vi "Frontend FPP.vi"() -> ()   [LabVIEW 2016]
panel:
  in  "Gate 2":T1={"Gate Start"=0.0, "Gate Stop"=2.0, "Gate Step (linear only)"=1.0, "Gate Compliance"=0.0001, "Gate PComp"=0.0, "Range mode"=0, "Range"=6} {"Range" max=11 scale=0.0..11.0; "Range mode" items=["Auto", "Limited", "Fixed"]; "Gate PComp" format="%^.2e"; "Gate Compliance" format="%^.2e"; "Gate Step (linear only)" format="%^.4e"; "Gate Stop" format="%^.4e"; "Gate Start" format="%^.4e"}
  in  "Drain":T2={"Drain Start"=0.0, "Drain Stop"=2.0, "Drain Compliance"=0.0001, "Drain Step"=1.0, "Drain PComp"=0.0, "Range mode"=0, "Range"=6} {"Range" max=11 scale=0.0..11.0; "Range mode" items=["Auto", "Limited", "Fixed"]; "Drain PComp" format="%^.2e"; "Drain Step" format="%^.4e"; "Drain Compliance" format="%^.2e"; "Drain Stop" format="%^.4e"; "Drain Start" format="%^.4e"}
  in  "Gate":T3={"Gate Start"=0.0, "Gate Stop"=2.0, "Gate Step"=1.0, "Gate Compliance"=0.0001, "Gate PComp"=0.0, "Range mode"=0, "Range"=6} {"Range" max=11 scale=0.0..11.0; "Range mode" items=["Auto", "Limited", "Fixed"]; "Gate PComp" format="%^.2e"; "Gate Compliance" format="%^.2e"; "Gate Step" format="%^.4e"; "Gate Stop" format="%^.4e"; "Gate Start" format="%^.4e"}
  in  "Drain 2":T4={"Drain Start"=0.0, "Drain Stop"=2.0, "Drain Compliance"=0.0001, "Drain Step (linear only)"=1.0, "Drain PComp"=0.0, "Range mode"=0, "Range"=6} {"Range" max=11 scale=0.0..11.0; "Range mode" items=["Auto", "Limited", "Fixed"]; "Drain PComp" format="%^.2e"; "Drain Step (linear only)" format="%^.4e"; "Drain Compliance" format="%^.2e"; "Drain Stop" format="%^.4e"; "Drain Start" format="%^.4e"}
  in  "Timings":T5={"integration time"=0, "Short/Long integration time"=0.00064, "hold time (sec)"=0.0, "delay time (sec)"=0.0, "Step Time (0 disables)"=0.0, "sweep method"=0, "Pulse period"=0.005, "Base voltage"=0.0, "Pulse width"=0.0005} {"Pulse width" min=0.0005 max=0.1 step=0.0001 format="%.4f"; "Base voltage" format="%^.4e"; "Pulse period" min=0.005 max=1.0 step=0.0001 format="%.4f"; "sweep method" items=["Continuous", "Pulsed"]; "Step Time (0 disables)" format="%.2f"; "delay time (sec)" format="%.4f"; "hold time (sec)" format="%.4f"; "Short/Long integration time" format="%^.0e"; "integration time" scale=0.0..2.0}
  in  "Panel controls":T6={"Emergency Stop"=refnum, "OutputGraph Max"=1e-05, "Text/Graph (text=false)"=FALSE} {"OutputGraph Max" format="%.2e"}
  in  "Panel Controls":T7={"Emergency Stop"=refnum, "TransGraph Max"=1e-05, "Text/Graph (text=false)"=FALSE} {"TransGraph Max" format="%.2e"}
  in  "Tab Control":enum32{"Characteristics", "Other parameters"}(tab)
  out "XY Graph 2":cluster{"Y data in":dbl[], "X data in":dbl[]}[](graph)
  in  "Integration time (long)":dbl=0.32 min=0.04 max=2.0 step=0.02 format="%.2f"
  in  "Integration time (short)":dbl=0.00064 min=8e-05 max=0.00192 step=8e-05 format="%^.0e"
  in  "Drain Range":u8(slide)=6 max=11 scale=0.0..11.0
  in  "Drain Range mode":u16(ring) items=["Auto", "Limited", "Fixed"]
  in  "Gate Range":u8(slide)=6 max=11 scale=0.0..11.0
  in  "Gate Range mode":u16(ring) items=["Auto", "Limited", "Fixed"]
  in  "Sampling mode":u32(slide) scale=0.0..4.0
  in  "Number of Samples":i32=500 min=0 step=1
  in  "Time":dbl=240.0 min=0.0 format="%.2f"
  in  "Drain":dbl=-10.0 min=-100.0 max=100.0 format="%.2f"
  in  "Gate":dbl=-60.0 min=-100.0 max=100.0 format="%.2f"
  in  "sweep method":u16(ring) items=["Continuous", "Pulsed"]
  out "Id":dbl format="%.2e"
  out "Ig":dbl format="%.2e"
  in  "Sweep Start":bool caption="Sweep start"
  in  "Interrupt run":bool
  in  "Running":bool
  out "Path":path
  in  "integration time":u32(slide)=1 max=2 step=1 scale=0.0..2.0
  in  "sweep mode":u16(ring)=1 items=["Single", "Double"]
  in  "Transfer Start":bool
  in  "Output Start":bool
  in  "Drain: Step":dbl=-1.0 min=-100.0 max=100.0 format="%.2f"
  in  "Drain: Stop":dbl=-60.0 min=-100.0 max=100.0 format="%.2f"
  in  "Drain:Start":dbl min=-100.0 max=100.0 format="%.2f"
  in  "Gate: Step":dbl=-20.0 min=-100.0 max=100.0 format="%.2f"
  in  "Gate: Stop":dbl=-60.0 min=-100.0 max=100.0 format="%.2f"
  in  "Gate: Start":dbl min=-100.0 max=100.0 format="%.2f"
  out "XY Graph":cluster{"Y data in":dbl[], "X data in":dbl[]}[](graph)
  in  "Drain: Compliance":dbl=0.001 min=1e-12 max=0.02 format="%.8f"
  in  "Gate: Compliance":dbl=0.001 min=1e-12 max=0.02 format="%.8f"
  in  "Drain: Step":dbl=-5.0 min=-100.0 max=100.0 format="%.2f"
  in  "Drain: Stop":dbl=-10.0 min=-100.0 max=100.0 format="%.2f"
  in  "Drain:Start":dbl=-5.0 min=-100.0 max=100.0 format="%.2f"
  in  "Gate: Step":dbl=-1.0 min=-100.0 max=100.0 format="%.2f"
  in  "Gate: Stop":dbl=-60.0 min=-100.0 max=100.0 format="%.2f"
  in  "Gate: Start":dbl=10.0 min=-100.0 max=100.0 format="%.2f"
  in  "Pulse width":dbl=0.0005 min=0.0005 max=0.1 step=0.0001 format="%.4f"
  in  "Base voltage":dbl min=-100.0 max=100.0 format="%.2f"
  in  "Pulse period":dbl=0.005 min=0.005 max=1.0 step=0.0001 format="%.4f"
  in  "Drain Power Compliance":dbl min=0.0 max=1.0 format="%.2f"
  in  "Gate Power\nCompliance":dbl min=0.0 max=1.0 format="%.2f"
  in  "OutputGraph Max":dbl=1e-05 format="%.2e"
  in  "TransGraph Max":dbl=1e-05 format="%.2e"
  in  "SPA Display":bool
  in  "Step delay /s":dbl min=0.0 max=1.0 format="%.2f"
  in  "hold time /s":dbl min=0.0 max=655.35 step=0.01 format="%.2f"
  in  "delay time /s":dbl min=0.0 max=65.535 step=0.0001 format="%.2f"
  in  "Decimal places in header":i8=1
  out "error out":errorcluster
  # "Transfer Characteristics"
  # "Stress Measurements"
  # "V"
  # "V"
  # "V"
  # "Gate"
  # "V"
  # "V"
  # "V"
  # "V"
  # "Drain"
  # "V"
  # "s"
  # "Output Characteristics"
  # "V"
  # "V"
  # "V"
  # "Gate"
  # "V"
  # "V"
  # "Drain"
  # "V"
  # "For Four Point Probe measurements ONLY!"
  # "SMU1 = Probe 1\nSMU2 = Drain\nSMU3 = Gate\nSMU4 = Probe 2\nVSU1 = Source"
  # "A"
  # "A"
  # "Vp1"
  # "Vp2"
  # "s"
  # "Pulsed mode settings"
  # "s"
  # "NOTE - THIS OVERRIDES THE COMPLIANCE VALUES!"
  # "A"
  # "A"
  # "Enter max power in Watts (max 1W)"
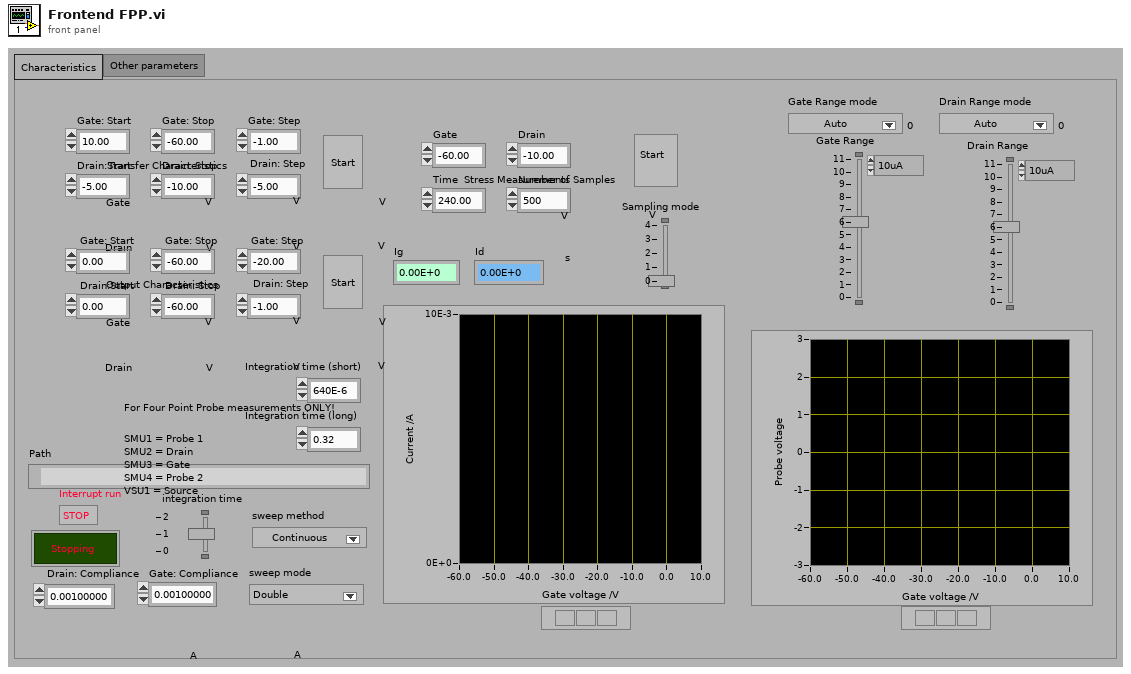
[diagram p1: front panel]
types:
  T1 = cluster{"Gate Start":dbl, "Gate Stop":dbl, "Gate Step (linear only)":dbl, "Gate Compliance":dbl, "Gate PComp":dbl, "Range mode":u16, "Range":u8}
  T2 = cluster{"Drain Start":dbl, "Drain Stop":dbl, "Drain Compliance":dbl, "Drain Step":dbl, "Drain PComp":dbl, "Range mode":u16, "Range":u8}
  T3 = cluster{"Gate Start":dbl, "Gate Stop":dbl, "Gate Step":dbl, "Gate Compliance":dbl, "Gate PComp":dbl, "Range mode":u16, "Range":u8}
  T4 = cluster{"Drain Start":dbl, "Drain Stop":dbl, "Drain Compliance":dbl, "Drain Step (linear only)":dbl, "Drain PComp":dbl, "Range mode":u16, "Range":u8}
  T5 = cluster{"integration time":u32, "Short/Long integration time":dbl, "hold time (sec)":dbl, "delay time (sec)":dbl, "Step Time (0 disables)":dbl, "sweep method":u16, "Pulse period":dbl, "Base voltage":dbl, "Pulse width":dbl}
  T6 = cluster{"Emergency Stop":refnum<vi>, "OutputGraph Max":dbl, "Text/Graph (text=false)":bool}
  T7 = cluster{"Emergency Stop":refnum<vi>, "TransGraph Max":dbl, "Text/Graph (text=false)":bool}
  T8 = cluster{"V2 Start":dbl, "V2 Step":dbl, "Number of points":i32}
  T9 = enum16{"open", "replace", "create", "open or create", "replace or create", "replace or create with confirmation"}
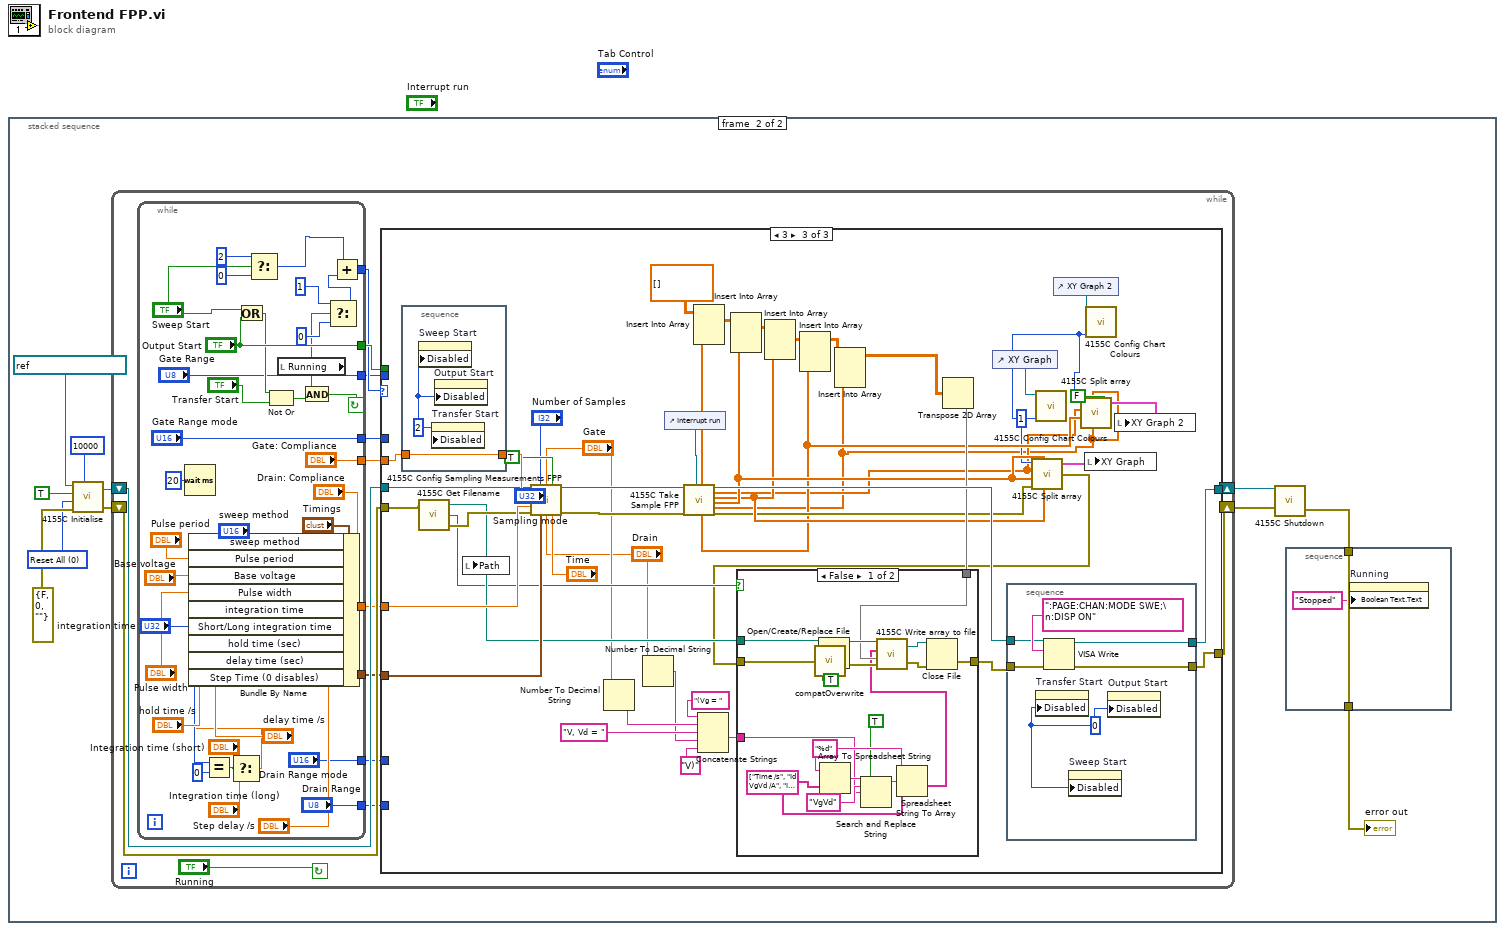
[diagram p0: block diagram]
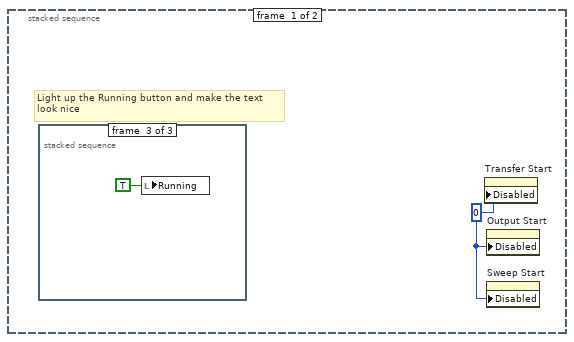
[diagram p2: hidden frame]
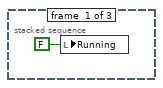
[diagram p3: hidden frame]
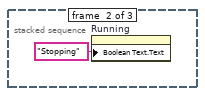
[diagram p4: hidden frame]
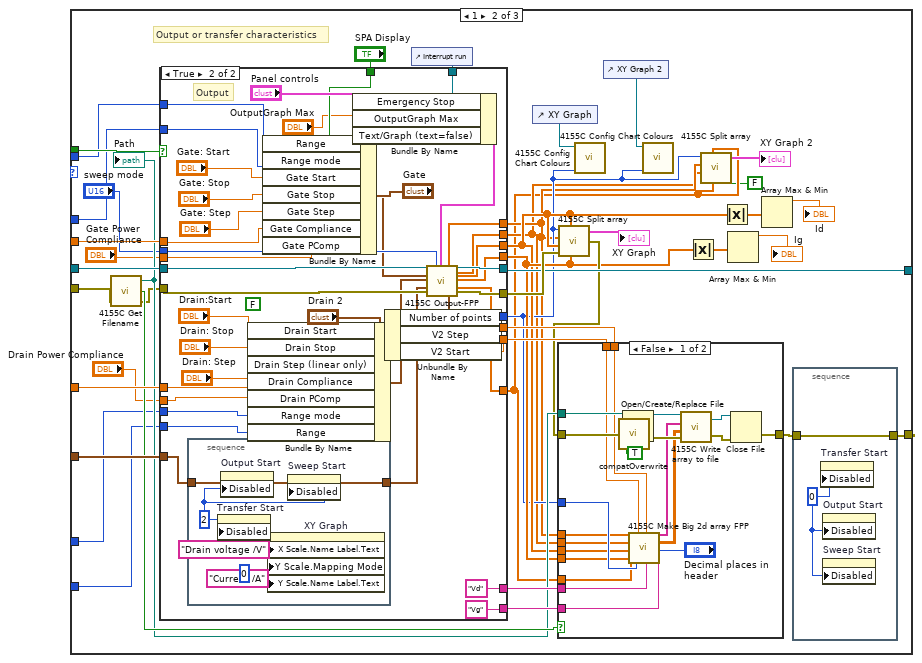
[diagram p6: hidden frame]
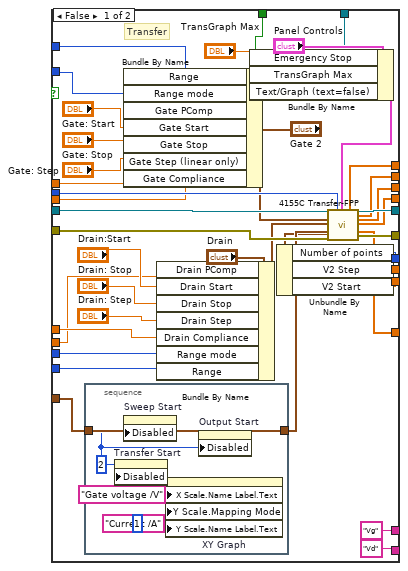
[diagram p8: hidden frame]
diagram:
  n1 = stacked-sequence {
    frame #0 {
      w1 = u8 0 ("Disabled")
      # "Light up the Running button and make the text\nlook nice"
      n2 = stacked-sequence {
        frame #0 {
          n3 = local write "Running"(FALSE ("Running")) -> ()
        }
        frame #1 {
          n4 = property on="Running" class="Bool (strict)"("Boolean Text.Text"="Stopping") -> ()  [unwired: 2 in, 2 out]
        }
        frame #2 {
          (unwired) FALSE ("Running")
          n5 = local write "Running"(TRUE ("Running")) -> ()
        }
      }
      n6 = property on="Transfer Start" class="Bool (strict)"("Disabled"=w1) -> ()  [unwired: 2 in, 2 out]
      n7 = property on="Output Start" class="Bool (strict)"("Disabled"=w1) -> ()  [unwired: 2 in, 2 out]
      n8 = property on="Sweep Start" class="Bool (strict)"("Disabled"=w1) -> ()  [unwired: 2 in, 2 out]
    }
    frame #1 {
      w11 = u16 0 items=["Reset All", "Partial reset"] ("Type of reset")
      n9 = call "4155C Initialise.vi"("VISA resource name in"=refnum<visa-resource-name> "GPIB0::14::INSTR", "Reset"=TRUE, "Type of reset"=w11, "error in (no error)"=errorcluster {"status"=FALSE, "code"=0, "source"=""}, "VISA Timeout Value"=u32 10000) -> ("VISA Resource Name out"=w10:refnum<visa-resource-name>, "error out"=w9:errorcluster)
      n10 = while {
        shift-left: w10 -> [w24]
        shift-right: [w26] -> w5
        shift-left: w9 -> [w25]
        shift-right: [w27] -> w6
        stop <- "Running" continue-if-true
        n11 = while {
          tunnel: ["Gate Range"] -> w16
          tunnel: ["Gate Range mode"] -> w17
          tunnel: ["Drain Range"] -> w18
          tunnel: ["Drain Range mode"] -> w19
          tunnel: ["Drain: Compliance"] -> w20
          tunnel: [w49] -> w21
          tunnel: ["Gate: Compliance"] -> w22
          tunnel: [w55] -> w23
          tunnel: ["Output Start"] -> w28
          stop <- w64 continue-if-true
          n12 = Wait (ms)(milliseconds to wait=u32 20) -> ()  [unwired: 1 out]
          n13 = Equal?(x="integration time", y=u32 0) -> (x = y?=w46:bool)
          n14 = Select(t="Integration time (short)", s=w46, f="Integration time (long)") -> (s? t:f=w43:dbl)
          n15 = Bundle By Name(cluster="Timings", "sweep method"="sweep method", "Pulse period"="Pulse period", "Base voltage"="Base voltage", "Pulse width"="Pulse width", "integration time"="integration time", "Short/Long integration time"=w43, "hold time (sec)"="hold time /s", "delay time (sec)"="delay time /s", "Step Time (0 disables)"="Step delay /s") -> (w49:T5)
          n16 = Or(x="Sweep Start", y="Output Start") -> (x .or. y?=w61:bool)
          n17 = Select(t=i8 2, s="Sweep Start", f=i8 0) -> (s? t:f=w31:i8)
          n18 = Not Or(1:"Transfer Start", 2:w61) -> (0:w63:bool)
          n19 = local read "Running"() -> (w58:bool)
          n20 = And(x=w58, y=w63) -> (x .and. y?=w64:bool)
          n21 = Select(t=i8 1, s=w58, f=i8 0) -> (s? t:f=w54:i8)
          n22 = Add(x=w31, y=w54) -> (x+y=w55:i8)
        }
        n23 = case shown="3" w23 {
          tunnel: w28 -> [_ w109 _]
          tunnel: w21 -> [_ w108 w266]
          tunnel: w22 -> [_ w107 w274]
          tunnel: w20 -> [_ w106 w270]
          tunnel: [w67 w97 w272] -> w27
          tunnel: [w66 w100 w273] -> w26
          tunnel: w25 -> [w67 w91 w261]
          tunnel: w24 -> [w66 w99 w260]
          tunnel: w19 -> [_ w81 _]
          tunnel: w18 -> [_ w80 _]
          tunnel: w17 -> [_ w79 _]
          tunnel: w16 -> [_ w78 _]
          frame 0, Default {
            # "Someone's deselected the running button so just shutdown..."
          }
          frame 1 {
            # "Output or transfer characteristics"
            n24 = call "4155C Get Filename.vi"("error in (no error)"=w91) -> ("error out"=w90:errorcluster, "cancelled"=w96:bool, "path"=w95:path)  [unwired: 2 in]
            "Path" <- w95
            n25 = control-ref of="Interrupt run"() -> (w92:refnum<vi>)
            n26 = case shown="True" w109 {
              tunnel: w99 -> [w161 w207]
              tunnel: w90 -> [w160 w206]
              tunnel: w108 -> [w164 w212]
              tunnel: w107 -> [w170 w219]
              tunnel: w106 -> [w175 w218]
              tunnel: "sweep mode" -> [w169 w217]
              tunnel: [w137 w185] -> w71
              tunnel: [w136 w184] -> w70
              tunnel: [w139 w183] -> w77
              tunnel: [w138 w182] -> w82
              tunnel: [w168 w216] -> w100
              tunnel: [w167 w215] -> w105
              tunnel: [w140 w188] -> w72
              tunnel: [w141 w187] -> w103
              tunnel: [w142 w186] -> w104
              tunnel: ["Vg" "Vd"] -> w102
              tunnel: ["Vd" "Vg"] -> w101
              tunnel: w92 -> [w158 w205]
              tunnel: "SPA Display" -> [w157 w203]
              tunnel: "Drain Power Compliance" -> [w153 w200]
              tunnel: "Gate Power\nCompliance" -> [w154 w199]
              tunnel: w81 -> [w145 w193]
              tunnel: w80 -> [w144 w192]
              tunnel: w79 -> [w146 w191]
              tunnel: w78 -> [w147 w190]
              tunnel: [w135 w181] -> w69
              frame False {
                # "Transfer"
                n27 = stacked-sequence {
                  tunnel: w164 -> [w179]
                  tunnel: [w179] -> w152
                  frame #0 {
                    w177 = u8 2 ("Disabled")
                    n28 = property on="Transfer Start" class="Bool (strict)"("Disabled"=w177) -> ()  [unwired: 2 in, 2 out]
                    n29 = property on="Sweep Start" class="Bool (strict)"("Disabled"=w177) -> ()  [unwired: 2 in, 2 out]
                    n30 = property on="XY Graph" class="XYGraph (strict)"("X Scale.Name Label.Text"="Gate voltage /V", "Y Scale.Mapping Mode"=u8 1, "Y Scale.Name Label.Text"="Current /A") -> ()  [unwired: 2 in, 2 out]
                    n31 = property on="Output Start" class="Bool (strict)"("Disabled"=w177) -> ()  [unwired: 2 in, 2 out]
                  }
                }
                n32 = Bundle By Name(cluster="Gate 2", "Range"=w147, "Range mode"=w146, "Gate PComp"=w154, "Gate Start"="Gate: Start", "Gate Stop"="Gate: Stop", "Gate Step (linear only)"="Gate: Step", "Gate Compliance"=w170) -> (w148:T1)
                n33 = Bundle By Name(cluster="Drain", "Drain PComp"=w153, "Drain Start"="Drain:Start", "Drain Stop"="Drain: Stop", "Drain Step"="Drain: Step", "Drain Compliance"=w175, "Range mode"=w145, "Range"=w144) -> (w150:T2)
                n34 = Bundle By Name(cluster="Panel Controls", "Emergency Stop"=w158, "TransGraph Max"="TransGraph Max", "Text/Graph (text=false)"=w157) -> (w155:T7)
                n35 = call "4155C Transfer-FPP.vi"("VISA resource name in"=w161, "Gate"=w148, "Drain"=w150, "Timings"=w152, "error in (no error)"=w160, "sweep mode"=w169, "Panel Controls"=w155) -> ("VG"=w137:dbl[], "Outparams"=w143:T8, "VISA Resource Name out"=w168:refnum<visa-resource-name>, "Vprobe2"=w136:dbl[], "ID"=w139:dbl[], "IG"=w138:dbl[], "Vprobe1"=w135:dbl[], "error out"=w167:errorcluster)  [unwired: 13 in]
                n36 = Unbundle By Name(w143) -> ("Number of points"=w140:i32, "V2 Step"=w141:dbl, "V2 Start"=w142:dbl)
              }
              frame True {
                (unwired) FALSE ("Logarithmic")
                # "Output"
                n37 = stacked-sequence {
                  tunnel: w212 -> [w225]
                  tunnel: [w225] -> w198
                  frame #0 {
                    w223 = u8 2 ("Disabled")
                    n38 = property on="Transfer Start" class="Bool (strict)"("Disabled"=w223) -> ()  [unwired: 2 in, 2 out]
                    n39 = property on="Output Start" class="Bool (strict)"("Disabled"=w223) -> ()  [unwired: 2 in, 2 out]
                    n40 = property on="XY Graph" class="XYGraph (strict)"("X Scale.Name Label.Text"="Drain voltage /V", "Y Scale.Mapping Mode"=u8 0, "Y Scale.Name Label.Text"="Current /A") -> ()  [unwired: 2 in, 2 out]
                    n41 = property on="Sweep Start" class="Bool (strict)"("Disabled"=w223) -> ()  [unwired: 2 in, 2 out]
                  }
                }
                n42 = Bundle By Name(cluster="Drain 2", "Drain Start"="Drain:Start", "Drain Stop"="Drain: Stop", "Drain Step (linear only)"="Drain: Step", "Drain Compliance"=w218, "Drain PComp"=w200, "Range mode"=w193, "Range"=w192) -> (w196:T4)
                n43 = Bundle By Name(cluster="Gate", "Range"=w190, "Range mode"=w191, "Gate Start"="Gate: Start", "Gate Stop"="Gate: Stop", "Gate Step"="Gate: Step", "Gate Compliance"=w219, "Gate PComp"=w199) -> (w194:T3)
                n44 = Bundle By Name(cluster="Panel controls", "Emergency Stop"=w205, "OutputGraph Max"="OutputGraph Max", "Text/Graph (text=false)"=w203) -> (w201:T6)
                n45 = call "4155C Output-FPP.vi"("VISA resource name in"=w207, "Gate"=w194, "Drain"=w196, "Timings"=w198, "error in (no error)"=w206, "sweep mode"=w217, "Panel controls"=w201) -> ("VD"=w185:dbl[], "Outparams"=w189:T8, "VISA Resource Name out"=w216:refnum<visa-resource-name>, "Vprobe2"=w184:dbl[], "ID"=w183:dbl[], "IG"=w182:dbl[], "Vprobe1"=w181:dbl[], "error out"=w215:errorcluster)  [unwired: 13 in]
                n46 = Unbundle By Name(w189) -> ("Number of points"=w188:i32, "V2 Step"=w187:dbl, "V2 Start"=w186:dbl)
              }
            }
            n47 = control-ref of="XY Graph"() -> (w93:refnum<vi>)
            n48 = call "4155C Split array.vi"("Number of VAR2 steps"=w72, "Y2 data in"=w77, "X data in"=w71, "Y1 data in"=w77, "Y3 data in"=w82, "error in (no error)"=w105) -> ("Array of clusters"=→"XY Graph":cluster{"Y data in":dbl[], "X data in":dbl[]}[], "error out"=w89:errorcluster)  [unwired: 1 in]
            n49 = case shown="False" w96 {
              tunnel: w89 -> [w132 w134]
              tunnel: [w127 w134] -> w98
              tunnel: w95 -> [w131 _]
              tunnel: w72 -> [w125 _]
              tunnel: w77 -> [w115 _]
              tunnel: w71 -> [w117 _]
              tunnel: w70 -> [w116 _]
              tunnel: w82 -> [w114 _]
              tunnel: w104 -> [w119 _]
              tunnel: w103 -> [w120 _]
              tunnel: w102 -> [w124 _]
              tunnel: w101 -> [w123 _]
              tunnel: w69 -> [w113 _]
              frame False {
                n50 = call <vilib>:"compatOverwrite.vi"("overwrite (F)"=TRUE) -> ("overwrite?"=w112:T9)
                n51 = Open/Create/Replace File(file path (use dialog)=w131, error in=w132, operation (0:open)=w112) -> (refnum out=w129:refnum<file>, error out=w130:errorcluster)  [unwired: 3 in, 1 out]
                n52 = call "4155C Make Big 2d array FPP.vi"("1D Var1"=w117, "1d ID"=w115, "1d Vp2"=w116, "1d IG"=w114, "1d Vp1"=w113, "VAR2 START"=w119, "Number of VAR2 steps"=w125, "VAR2 STEP"=w120, "VAR1 Name"=w124, "Decimal places in header"="Decimal places in header", "VAR2 Name"=w123) -> ("Header array"=w121:string[], "Data array"=w122:dbl[][])  [unwired: 15 in]
                n53 = call "4155C Write array to file.vi"("Byte Stream File Refnum"=w129, "Header"=w121, "Data Array"=w122, "error in (no error)"=w130) -> ("dup refnum"=w126:refnum<file>, "error out"=w128:errorcluster)  [unwired: 1 in]
                n54 = Close File(refnum=w126, error in=w128) -> (error out=w127:errorcluster)  [unwired: 1 out]
              }
              frame True {
              }
            }
            n55 = call "4155C Config Chart Colours.vi"("Numeric"=w72, "XY Graph 2"=w93) -> ()  [unwired: 6 in]
            n56 = control-ref of="XY Graph 2"() -> (w74:refnum<vi>)
            n57 = call "4155C Config Chart Colours.vi"("Numeric"=w72, "XY Graph 2"=w74) -> ()  [unwired: 6 in]
            n58 = Absolute Value(x=w82) -> (abs(x)=w84:dbl[])
            n59 = call "4155C Split array.vi"("Number of VAR2 steps"=w72, "Y2 data in"=w69, "X data in"=w71, "Y1 data in"=w70, "Y3 data in"=w69, "Absolute val?"=FALSE) -> ("Array of clusters"=→"XY Graph 2":cluster{"Y data in":dbl[], "X data in":dbl[]}[])  [unwired: 1 in, 1 out]
            n60 = Absolute Value(x=w77) -> (abs(x)=w83:dbl[])
            n61 = Array Max & Min(array=w84) -> (max value=→"Ig":dbl)  [unwired: 3 out]
            n62 = Array Max & Min(array=w83) -> (max value=→"Id":dbl)  [unwired: 3 out]
            n63 = stacked-sequence {
              tunnel: w98 -> [w111]
              tunnel: [w111] -> w97
              frame #0 {
                w110 = u8 0 ("Disabled")
                n64 = property on="Transfer Start" class="Bool (strict)"("Disabled"=w110) -> ()  [unwired: 2 in, 2 out]
                n65 = property on="Output Start" class="Bool (strict)"("Disabled"=w110) -> ()  [unwired: 2 in, 2 out]
                n66 = property on="Sweep Start" class="Bool (strict)"("Disabled"=w110) -> ()  [unwired: 2 in, 2 out]
              }
            }
          }
          frame 3 {
            w230 = 1 ("Numeric")
            n67 = stacked-sequence {
              tunnel: w274 -> [w301]
              tunnel: [w301] -> w271
              frame #0 {
                w300 = u8 2 ("Disabled")
                n68 = property on="Sweep Start" class="Bool (strict)"("Disabled"=w300) -> ()  [unwired: 2 in, 2 out]
                n69 = property on="Transfer Start" class="Bool (strict)"("Disabled"=w300) -> ()  [unwired: 2 in, 2 out]
                n70 = property on="Output Start" class="Bool (strict)"("Disabled"=w300) -> ()  [unwired: 2 in, 2 out]
              }
            }
            n71 = call "4155C Get Filename.vi"("error in (no error)"=w261) -> ("error out"=w259:errorcluster, "cancelled"=w250:bool, "path"=w251:path)  [unwired: 2 in]
            n72 = local write "Path"(w251) -> ()
            n73 = call "4155C Config Sampling Measurements FPP.vi"("VISA session"=w260, "Num Points"="Number of Samples", "Vg"="Gate", "Display on/off"=TRUE, "Gate Compliance"=w271, "Sampling mode"="Sampling mode", "Drain Compliance"=w270, "error in (no error)"=w259, "Timings"=w266, "Vd"="Drain", "Sample time"="Time") -> ("dup VISA resource name"=w267:refnum<visa-resource-name>, "error out"=w268:errorcluster)  [unwired: 3 in]
            n74 = Number To Decimal String(number="Gate") -> (decimal integer string=w248:string)  [unwired: 1 in]
            n75 = Number To Decimal String(number="Drain") -> (decimal integer string=w246:string)  [unwired: 1 in]
            n76 = control-ref of="Interrupt run"() -> (w262:refnum<vi>)
            n77 = call "4155C Take Sample FPP.vi"("VISA resource name in"=w267, "error in (no error)"=w268, "Emergency Stop"=w262) -> ("Time"=w228:dbl[], "Vp1"=w232:dbl[], "VISA Resource Name out"=w269:refnum<visa-resource-name>, "Ig"=w240:dbl[], "Id"=w241:dbl[], "Vp2"=w227:dbl[], "error out"=w239:errorcluster)  [unwired: 10 in]
            n78 = Insert Into Array(array=dbl[][] [] ("Input Array"), new element=w228) -> (w258:dbl[][])  [unwired: 2 in]
            n79 = Concatenate Strings("(Vg = " ("Substring"), w248, "V, Vd = " ("Substring"), w246, "V)" ("Substring")) -> (w244:string)
            n80 = Insert Into Array(array=w258, new element=w241) -> (w257:dbl[][])  [unwired: 2 in]
            n81 = Insert Into Array(array=w257, new element=w240) -> (w256:dbl[][])  [unwired: 2 in]
            n82 = Insert Into Array(array=w256, new element=w232) -> (w254:dbl[][])  [unwired: 2 in]
            n83 = Insert Into Array(array=w254, new element=w227) -> (w234:dbl[][])  [unwired: 2 in]
            n84 = Transpose 2D Array(2D array=w234) -> (transposed array=w252:dbl[][])
            n85 = control-ref of="XY Graph"() -> (w243:refnum<vi>)
            n86 = call "4155C Split array.vi"("Number of VAR2 steps"=w230, "Y2 data in"=w241, "X data in"=w228, "Y1 data in"=w241, "Y3 data in"=w240, "error in (no error)"=w239) -> ("Array of clusters"=w242:cluster{"Y data in":dbl[], "X data in":dbl[]}[], "error out"=w238:errorcluster)  [unwired: 1 in]
            n87 = case shown="False" w250 {
              tunnel: w238 -> [w291 w293]
              tunnel: [w286 w293] -> w253
              tunnel: w251 -> [w290 _]
              tunnel: w252 -> [w284 _]
              tunnel: w244 -> [w276 _]
              frame False {
                w277 = string[] ["Time /s", "Id VgVd /A", "Ig VgVd /A", "Vp1 VgVd /V", "Vp2 VgVd /V"] ("Header")
                w281 = "%d" ("format string")
                n88 = call <vilib>:"compatOverwrite.vi"("overwrite (F)"=TRUE) -> ("overwrite?"=w275:T9)
                n89 = Open/Create/Replace File(file path (use dialog)=w290, error in=w291, operation (0:open)=w275) -> (refnum out=w288:refnum<file>, error out=w289:errorcluster)  [unwired: 3 in, 1 out]
                n90 = Array To Spreadsheet String(array=w277, 3:w281) -> (spreadsheet string=w283:string)  [unwired: 1 in]
                n91 = Search and Replace String(replace all?=TRUE ("replace all? (F)"), input string=w283, search string="VgVd", replace string=w276) -> (result string=w279:string)  [unwired: 4 in, 3 out]
                n92 = Spreadsheet String To Array(format string=w281, spreadsheet string=w279, array type (2D Dbl)=w277) -> (array=w278:string[])  [unwired: 1 in]
                n93 = call "4155C Write array to file.vi"("Byte Stream File Refnum"=w288, "Header"=w278, "Data Array"=w284, "error in (no error)"=w289) -> ("dup refnum"=w285:refnum<file>, "error out"=w287:errorcluster)  [unwired: 1 in]
                n94 = Close File(refnum=w285, error in=w287) -> (error out=w286:errorcluster)  [unwired: 1 out]
              }
              frame True {
              }
            }
            n95 = stacked-sequence {
              tunnel: [w296] -> w273
              tunnel: [w295] -> w272
              tunnel: w269 -> [w298]
              tunnel: w253 -> [w297]
              frame #0 {
                w294 = u8 0 ("Disabled")
                n96 = property on="Transfer Start" class="Bool (strict)"("Disabled"=w294) -> ()  [unwired: 2 in, 2 out]
                n97 = VISA Write(VISA resource name=w298, write buffer=":PAGE:CHAN:MODE SWE;\n:DISP ON" ("write buffer (\"\")"), error in (no error)=w297) -> (VISA resource name out=w296:refnum<visa-resource-name>, error out=w295:errorcluster)  [unwired: 1 out]
                n98 = property on="Sweep Start" class="Bool (strict)"("Disabled"=w294) -> ()  [unwired: 2 in, 2 out]
                n99 = property on="Output Start" class="Bool (strict)"("Disabled"=w294) -> ()  [unwired: 2 in, 2 out]
              }
            }
            n100 = call "4155C Config Chart Colours.vi"("Numeric"=w230, "XY Graph 2"=w243) -> ()  [unwired: 6 in]
            n101 = control-ref of="XY Graph 2"() -> (w233:refnum<vi>)
            n102 = call "4155C Split array.vi"("Number of VAR2 steps"=w230, "Y2 data in"=w227, "X data in"=w228, "Y1 data in"=w232, "Y3 data in"=w227, "Absolute val?"=FALSE) -> ("Array of clusters"=w231:cluster{"Y data in":dbl[], "X data in":dbl[]}[])  [unwired: 1 in, 1 out]
            n103 = local write "XY Graph"(w242) -> ()
            n104 = call "4155C Config Chart Colours.vi"("Numeric"=w230, "XY Graph 2"=w233) -> ()  [unwired: 6 in]
            n105 = local write "XY Graph 2"(w231) -> ()
          }
        }
      }
      n106 = call "4155C Shutdown.vi"("VISA resource name in"=w5, "error in (no error)"=w6) -> ("error out"=w8:errorcluster)  [unwired: 4 in]
      n107 = stacked-sequence {
        tunnel: w8 -> [w303]
        tunnel: [w303] -> w7
        frame #0 {
          n108 = property on="Running" class="Bool (strict)"("Boolean Text.Text"="Stopped") -> ()  [unwired: 2 in, 2 out]
        }
      }
      "error out" <- w7
    }
  }
